vi "Load Top-Level VI.vi"() -> ()   [LabVIEW 2009]
panel:
  out "error out":errorcluster
  # "Loading User Interface, Please Wait..."
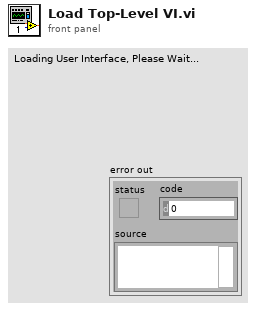
[diagram p1: front panel]
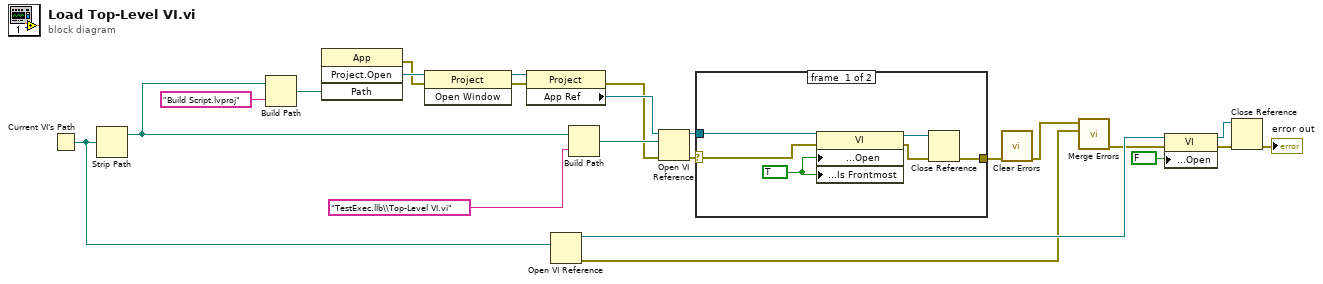
[diagram p0: block diagram]
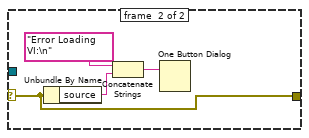
[diagram p2: hidden frame]
diagram:
  n1 = Current VI's Path() -> (path=w13:path)
  n2 = Strip Path(path=w13) -> (stripped path=w11:path)  [unwired: 1 out]
  n3 = Build Path(base path=w11, name or relative path="Build Script.lvproj") -> (appended path=w9:path)
  n4 = invoke class="App" method="Project.Open"("Path"=w9) -> (error out=w2:errorcluster, "Project:Open"=w4:refnum<vi>)  [unwired: 3 in, 2 out]
  n5 = invoke class="Project" method="Open Window"(reference=w4, error in=w2) -> (reference out=w3:refnum<vi>, error out=w1:errorcluster)  [unwired: 1 in, 1 out]
  n6 = property class="Project"(reference=w3, error in=w1) -> (error out=w8:errorcluster, "App Ref"=w12:refnum<vi>)  [unwired: 1 out]
  n7 = Open VI Reference(vi path=w13) -> (vi reference=w17:refnum<vi>, error out=w6:errorcluster)  [unwired: 1 in, 4 out]
  n8 = Build Path(base path=w11, name or relative path="TestExec.llb\\Top-Level VI.vi") -> (appended path=w22:path)
  n9 = Open VI Reference(application reference (local)=w12, vi path=w22, error in (no error)=w8) -> (vi reference=w21:refnum<vi>, error out=w20:errorcluster)  [unwired: 3 out]
  n10 = case shown="No Error" w20 {
    selector: w20 -> [w25 w30]
    tunnel: w21 -> [w29 _]
    tunnel: [w24 w30] -> w19
    frame #0 {
      w28 = TRUE ("Front Panel Window:Open")
      n11 = property class="VI"(reference=w29, error in=w25, "Front Panel Window:Open"=w28, "Front Panel Window:Is Frontmost"=w28) -> (reference out=w27:refnum<vi>, error out=w26:errorcluster)
      n12 = Close Reference(reference=w27, error in (no error)=w26) -> (error out=w24:errorcluster)
    }
    frame #1 {
      n13 = Unbundle By Name(w30) -> ("source"=w33:string)
      n14 = Concatenate Strings("Error Loading VI:\n" ("string"), w33) -> (w31:string)
      n15 = One Button Dialog(message=w31) -> ()  [unwired: 2 out]
    }
  }
  n16 = call <vilib>:"Clear Errors.vi"("error in (no error)"=w19) -> ("error out"=w7:errorcluster)  [unwired: 6 out]
  n17 = call <vilib>:"Merge Errors.vi"("error in 2 (no error)"=w6, "error in 1 (no error)"=w7) -> ("error out"=w5:errorcluster)  [unwired: 5 in]
  n18 = property class="VI"(reference=w17, error in=w5, "Front Panel Window:Open"=FALSE) -> (reference out=w15:refnum<vi>, error out=w16:errorcluster)
  n19 = Close Reference(reference=w15, error in (no error)=w16) -> (error out=→"error out":errorcluster)
